vi "Draw Steering Frame.vi"(4 "Side View Draw Area Size 2":T2, 6 "Top View Draw Area Size":T2, 8 "error in (no error)":errorcluster, 11 "ROV in":refnum<class "ROV Host.lvclass">) -> (0 "error out":errorcluster, 3 "ROV out":refnum<class "ROV Host.lvclass">, 5 "Side View":picture, 7 "Top View":picture)   [LabVIEW 2012, in "ROV Host.lvclass"]
uses:
  ROV Host.lvclass
  <vilib>/Utility/miscctls.llb/LVBoundsTypeDef.ctl
  <vilib>/robotics/Utilities/Visualization/Steering Visualization/Steering Picture/Draw Steering Frame Options.ctl
  ROV Host.lvclass/ROV Host.ctl
  <vilib>/robotics/Steering/Steering Frame/NI_Robotics_Steering Frame.lvclass/NI_Robotics_Steering Frame.ctl
  <vilib>/robotics/Steering/Steering Frame/Get Steering Frame Velocity from Wheels.vi
  <vilib>/robotics/Utilities/Visualization/Steering Visualization/Steering Picture/NI_Robotics_Steering Picture.lvlib
  <vilib>/robotics/Steering/Steering Frame/NI_Robotics_Steering Frame.lvclass
panel:
  in  "drawing options":T1={"draw wheel states?"=FALSE, "highlight wheel index"=-1, "pixels per unit"=50.0, "draw forward velocity?"=TRUE, "velocity scale"=1.0}
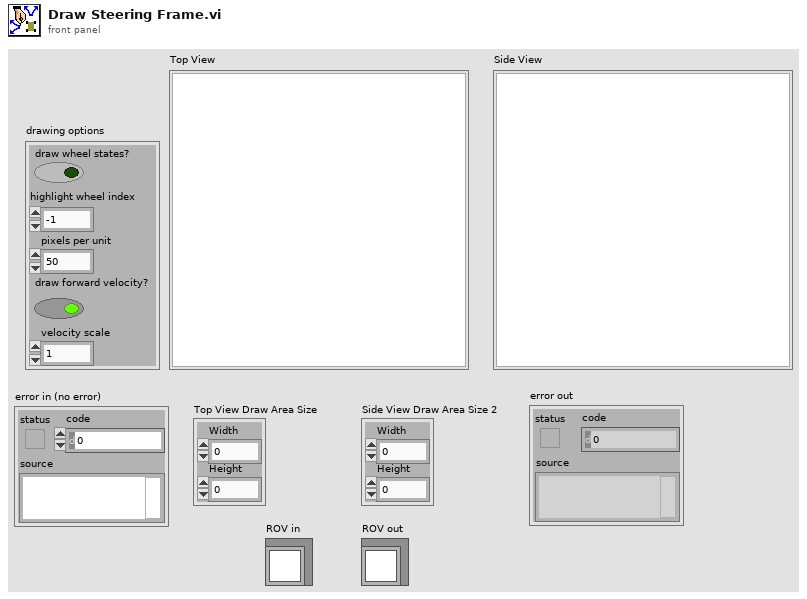
[diagram p1: front panel]
types:
  T1 = typedef "NI_Robotics_Steering Picture.lvlib/Draw Steering Frame Options.ctl" = cluster{"draw wheel states?":bool, "highlight wheel index":i32, "pixels per unit":dbl, "draw forward velocity?":bool, "velocity scale":dbl}
  T2 = typedef "LVBoundsTypeDef.ctl" = cluster{"Width":u32, "Height":u32}
  T3 = cluster{"x position":dbl, "y position":dbl, "angle (rad)":dbl}
  T4 = typedef "NI_Robotics_Steering Class Types.lvlib/Mecanum Steering Frame.ctl" = refnum<class "NI_Robotics_Mecanum Steering Frame.lvclass">
  T5 = typedef "NI_Robotics_Steering Class Types.lvlib/Differential Steering Frame.ctl" = refnum<class "NI_Robotics_Differential Steering Frame.lvclass">
  T6 = typedef "NI_Robotics_Wheel.lvclass/Wheel State.ctl" = cluster{"wheel name":string, "forward angular velocity":dbl, "caster angular velocity":dbl, "caster wheel angle (rad)":dbl, "steering angle (rad)":dbl}
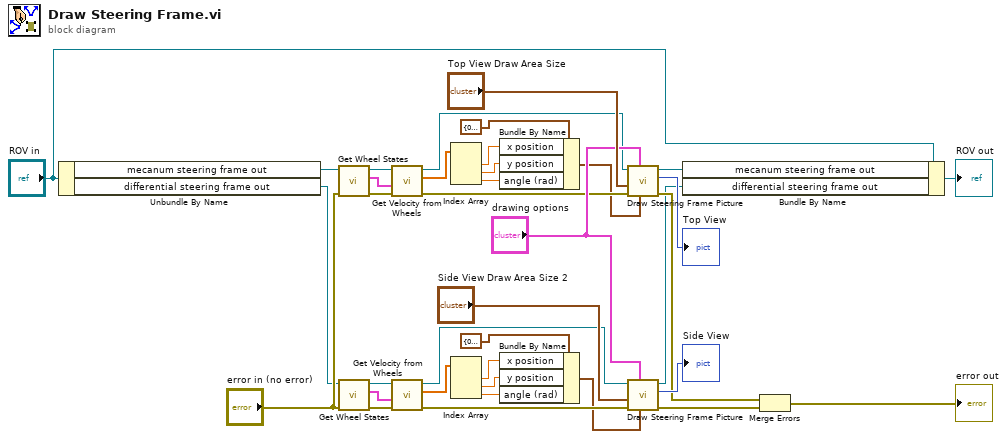
[diagram p0: block diagram]
diagram:
  n1 = Unbundle By Name("ROV in") -> ("mecanum steering frame out"=w4:T4, "differential steering frame out"=w3:T5)
  n2 = call <vilib>:"Get Wheel States.vi"("error in (no error)"="error in (no error)", "steering frame in"=w4) -> ("error out"=w7:errorcluster, "wheel states"=w9:T6[], "steering frame out"=w10:T4)  [unwired: 7 in]
  n3 = call <vilib>:"Get Wheel States.vi"("error in (no error)"="error in (no error)", "steering frame in"=w3) -> ("error out"=w11:errorcluster, "wheel states"=w13:T6[], "steering frame out"=w12:T5)  [unwired: 7 in]
  n4 = call-poly <vilib>:"Get Velocity from Wheels.vi"("error in (no error)"=w7, "acquired wheel states"=w9, "steering frame in"=w10) -> ("error out"=w29:errorcluster, "estimated steering frame velocity"=w14:dbl[], "steering frame out"=w27:T4)  [unwired: 5 in, 1 out]
  n5 = call-poly <vilib>:"Get Velocity from Wheels.vi"("error in (no error)"=w11, "acquired wheel states"=w13, "steering frame in"=w12) -> ("error out"=w28:errorcluster, "estimated steering frame velocity"=w23:dbl[], "steering frame out"=w26:T5)  [unwired: 5 in, 1 out]
  n6 = Index Array(array=w14) -> (element #1=w17:dbl, element #2=w18:dbl, element #3=w19:dbl)  [unwired: 3 in]
  n7 = Index Array(array=w23) -> (element #1=w22:dbl, element #2=w21:dbl, element #3=w20:dbl)  [unwired: 3 in]
  n8 = Bundle By Name(cluster=T3 {"x position"=0.0, "y position"=0.0, "angle (rad)"=0.0} ("steering frame position"), "x position"=w17, "y position"=w18, "angle (rad)"=w19) -> (w15:T3)
  n9 = Bundle By Name(cluster=T3 {"x position"=0.0, "y position"=0.0, "angle (rad)"=0.0} ("steering frame position"), "x position"=w22, "y position"=w21, "angle (rad)"=w20) -> (w24:T3)
  n10 = call <vilib>:"Draw Steering Frame Picture.vi"("steering frame position"=w15, "drawing options"="drawing options", "error in (no error)"=w29, "picture draw area size (pixels)"="Top View Draw Area Size", "steering frame in"=w27) -> ("error out"=w34:errorcluster, "picture out"=→"Top View":picture, "steering frame out"=w2:T4)  [unwired: 4 in]
  n11 = call <vilib>:"Draw Steering Frame Picture.vi"("steering frame position"=w24, "drawing options"="drawing options", "error in (no error)"=w28, "picture draw area size (pixels)"="Side View Draw Area Size 2", "steering frame in"=w26) -> ("error out"=w33:errorcluster, "picture out"=→"Side View":picture, "steering frame out"=w1:T5)  [unwired: 4 in]
  n12 = Bundle By Name(cluster="ROV in", "mecanum steering frame out"=w2, "differential steering frame out"=w1) -> (→"ROV out":refnum<class "ROV Host.lvclass">)
  n13 = Merge Errors(w34, w33) -> (→"error out":errorcluster)
